vi "Laser 1 FP handler L3.vi"(5 "VISA Resource":T3[](array[typedef]), 6 "Numeric":dbl[](array[numeric]), 7 "FP Ops":T1, 8 "Error in":errorcluster caption="Error in (no error)", 9 "Boolean":bool[](array[boolean]), 10 "I/p string(s)":string[](array[string]), 11 "UI elements cluster":T2) -> (0 "Error out":errorcluster, 2 "Read Wavelength":dbl, 3 "Ls1 User Controls 2":T4)   [LabVIEW 2020]
uses:
  Type Defs/Ls1 User Controls.ctl
  Serial Comms/Visa resource.ctl
  Typedefs/UI ctrl refs cluster.ctl
  Typedefs/Laser control knob.ctl
  Typedefs/Frame Size.ctl
  Typedefs/Plane Mode.ctl
  Typedefs/PMT control knob.ctl
  Typedefs/XY Stage_Move.ctl
  Typedefs/test_fpga_control.ctl
  Acquisition/Typedefs/Ref DAQ Param.ctl
  User Interface/Misc/Experiment Type.ctl
  User Interface/Misc/Biology Information.ctl
  Type Defs/Ls1 User Ops.ctl
panel:
  out "Array":errorcluster[](array[cluster])
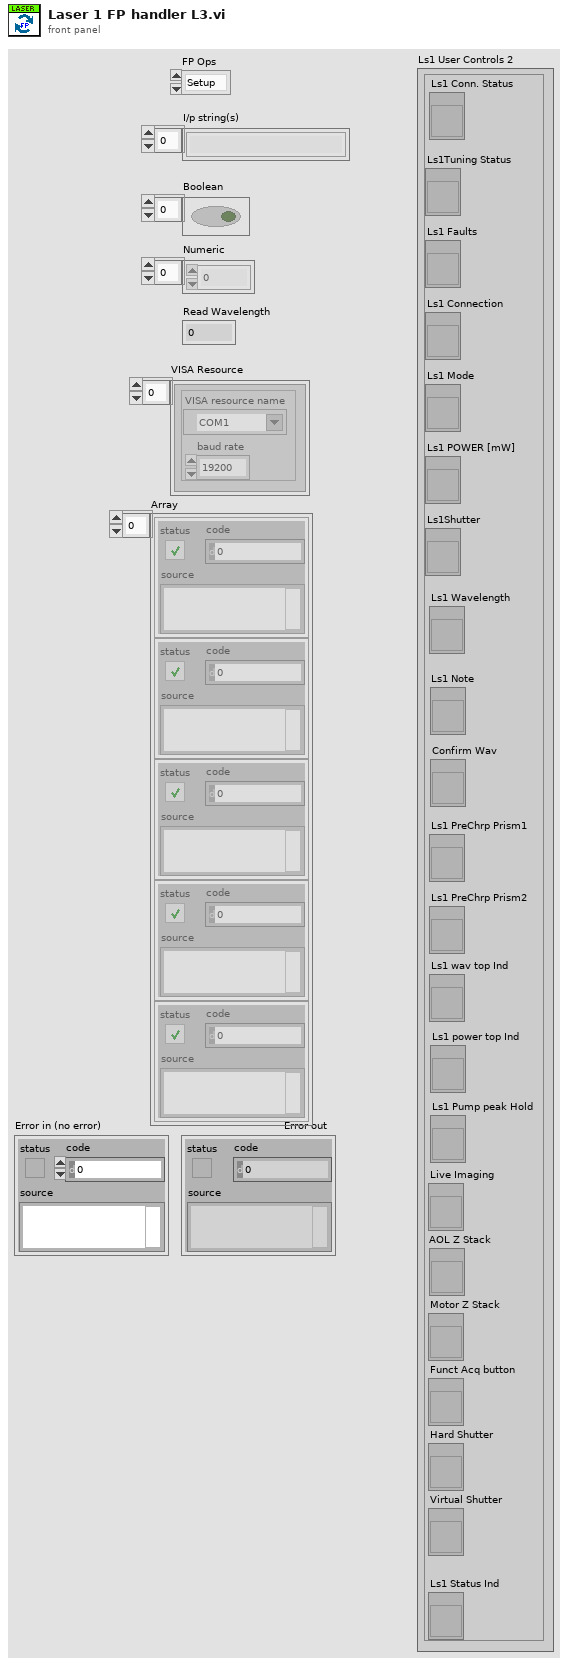
[diagram p1: front panel]
types:
  T1 = typedef "Ls1 User Ops.ctl" = enum16{"Setup", "Initialise", "Disable Controls", "Enable Controls", "Update Connection Info", "Update Laser Warning", "Update Laser status", "Update Laser status - sel", "Update Laser Wav.", "Update Laser Power", "Update prechiper settings", "Update Laser Note", "Update Shutter Status", "Close"}
  T2 = typedef "UI ctrl refs cluster.ctl" = cluster{"Top level VI path":path, "Top level VI ref":refnum<vi>, "User menu ref":refnum<k9>, "Sub Panel control":refnum<vi>, "Imaging Param Tab":refnum<vi>, "Occurrence-Start drivers":refnum<k4>, "Occurrence-Speed logging initialised":refnum<k4>, "Occurrence-XYZ stage initialised":refnum<k4>, "Exit button":refnum<vi>, "Status ind":refnum<vi>, "Set as origin":refnum<vi>, "Speed Logging":refnum<vi>, "Time Lapse":refnum<vi>, "Live Imaging":refnum<vi>, "AOL Z Stack":refnum<vi>, "Motor Z Stack":refnum<vi>, "Funct Acq button":refnum<vi>, "Hard Shutter":refnum<vi>, "Virtual Shutter":refnum<vi>, "Laser Power":refnum<vi>, "AOL Mode":refnum<vi>, "Frame Size":refnum<vi>, "Field of View":refnum<vi>, "Dwell Time":refnum<vi>, "Zoom":refnum<vi>, "AOL Z":refnum<vi>, "Objective":refnum<vi>, "Axis":refnum<vi>, "Paths & Names":refnum<vi>, "Experiment folder path (ind.)":refnum<vi>, "Last State (Ind.)":refnum<vi>, "Averages":refnum<vi>, "Angle (degrees)":refnum<vi>, "X centre":refnum<vi>, "Y centre":refnum<vi>, "Plane Mode":refnum<vi>, "# Planes":refnum<vi>, "Z Start":refnum<vi>, "Z Stop":refnum<vi>, "Z Step":refnum<vi>, "PMT 1":refnum<vi>, "PMT 2":refnum<vi>, "Stage XYZ Position":refnum<vi>, "Pockels@Z Start":refnum<vi>, "Pockels@Z Stop":refnum<vi>, "Obtain Z Start":refnum<vi>, "Obtain Z Stop":refnum<vi>, "Live stim.trig.period":refnum<vi>, "Live stim.trig.enable":refnum<vi>, "Movement Correction":refnum<vi>, "Load Reference Image":refnum<vi>, "XY Stage Move":refnum<vi>, "MovCor Cluster":refnum<vi>, "RefDAQParam":refnum<vi>, "Funct. Acq. Pockels Modulation":refnum<vi>, "Ref Laser Power":refnum<vi>, "Enable Video Recording":refnum<vi>, "Video Record-Live Imaging":refnum<vi>, "Video Record-Funct acq":refnum<vi>, "Reference Source":refnum<vi>, "AOL Z-stack Chirps Ready (ind)":refnum<vi>, "Target time between mov.cor. ref triggers (ms)":refnum<vi>, "Funct. Acq. Ref frame save":refnum<vi>, "Tracking button":refnum<vi>, "Show ref plots window":refnum<vi>, "Center freq ind (nm)":refnum<vi>, "Pickup mode (ind)":refnum<vi>, "Logging queue (ind)":refnum<vi>, "Back aperture power (ind.)":refnum<vi>, "Power after objective (ind.)":refnum<vi>, "Switch user":refnum<vi>, "Ls1 Conn. Status":refnum<vi>, "Ls1Tuning Status":refnum<vi>, "Ls1 Faults":refnum<vi>, "Ls1 Connection":refnum<vi>, "Ls1 Mode":refnum<vi>, "Ls1 POWER [mW]":refnum<vi>, "Ls1Shutter":refnum<vi>, "Ls1 Wavelength":refnum<vi>, "Ls1 Note":refnum<vi>, "Ls1 Confirm Wav":refnum<vi>, "Ls1 PreChrp Prism1":refnum<vi>, "Ls1 PreChrp Prism2":refnum<vi>, "Ls1 wav top Ind":refnum<vi>, "Ls1 power top Ind":refnum<vi>, "Ls1 Pump peak Hold":refnum<vi>, "Ls1 Status Ind":refnum<vi>, "Ls1 wav cancel":refnum<vi>, "Experiment Type":refnum<vi>, "Biology Information":refnum<vi>, "Camera recording status":refnum<vi>, "Optimise Obj. Pos.":refnum<vi>}
  T3 = typedef "Visa resource.ctl" = cluster{"VISA resource name":refnum<visa-resource-name>, "baud rate":u32}
  T4 = typedef "Ls1 User Controls.ctl" = cluster{"Ls1 Conn. Status":refnum<vi>, "Ls1Tuning Status":refnum<vi>, "Ls1 Faults":refnum<vi>, "Ls1 Connection":refnum<vi>, "Ls1 Mode":refnum<vi>, "Ls1 POWER [mW]":refnum<vi>, "Ls1Shutter":refnum<vi>, "Ls1 Wavelength":refnum<vi>, "Ls1 Note":refnum<vi>, "Confirm Wav":refnum<vi>, "Ls1 PreChrp Prism1":refnum<vi>, "Ls1 PreChrp Prism2":refnum<vi>, "Ls1 wav top Ind":refnum<vi>, "Ls1 power top Ind":refnum<vi>, "Ls1 Pump peak Hold":refnum<vi>, "Live Imaging":refnum<vi>, "AOL Z Stack":refnum<vi>, "Motor Z Stack":refnum<vi>, "Funct Acq button":refnum<vi>, "Hard Shutter":refnum<vi>, "Virtual Shutter":refnum<vi>, "Ls1 Status Ind":refnum<vi>}
  T5 = enum8{"Enabled", "Disabled", "Disabled and Grayed Out"}
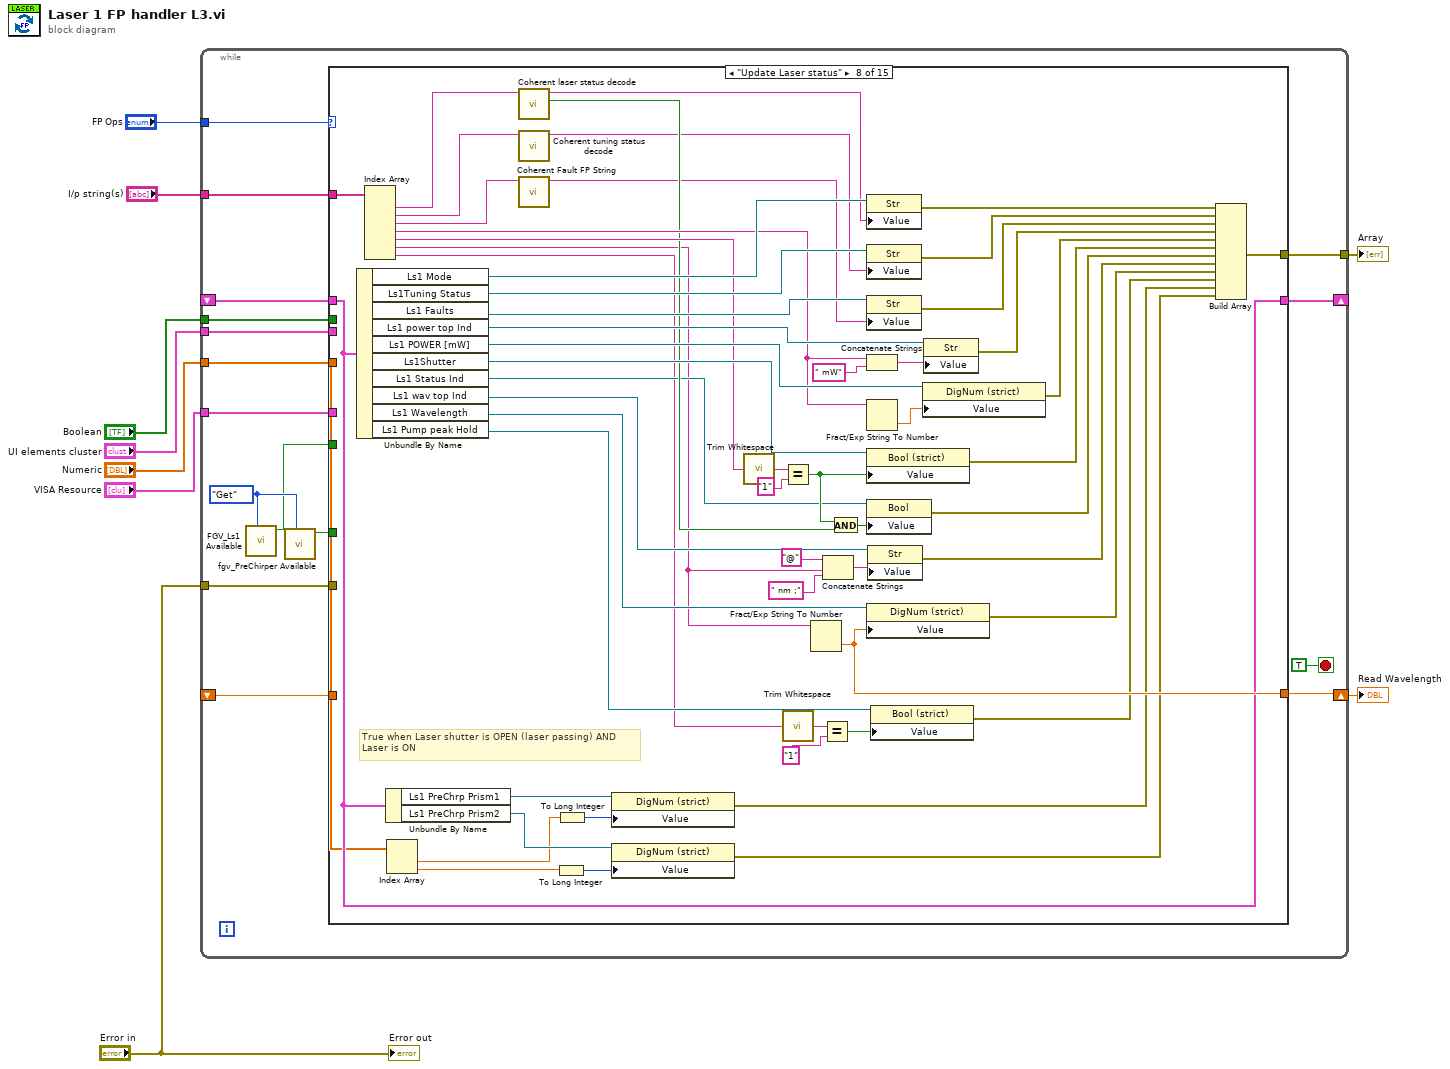
[diagram p0: block diagram]
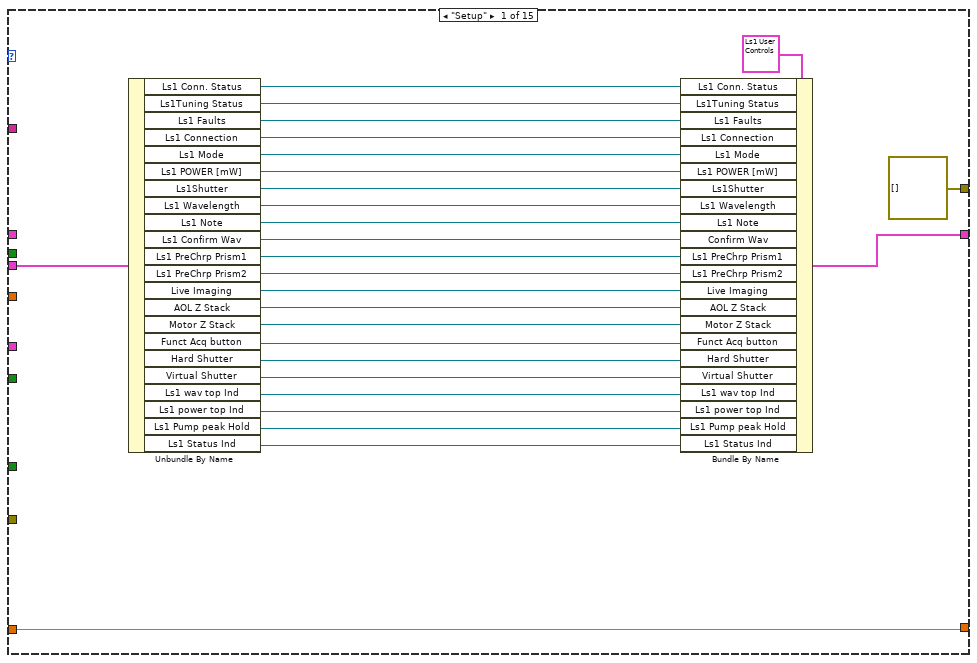
[diagram p2: hidden frame]
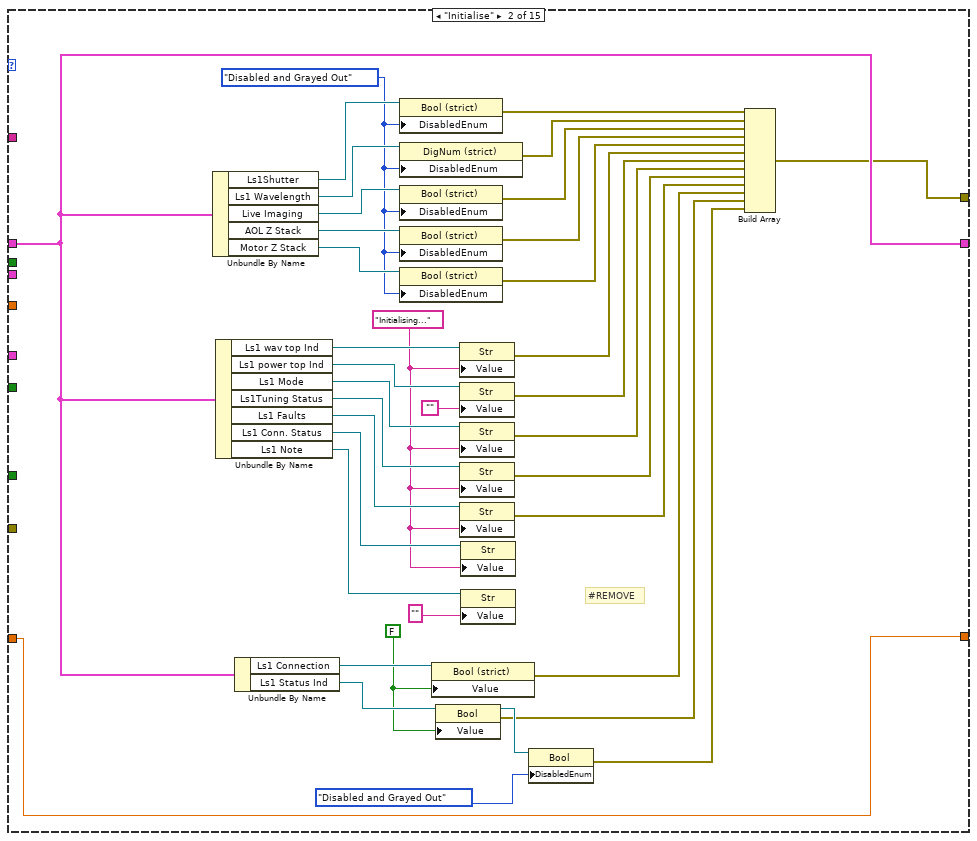
[diagram p3: hidden frame]
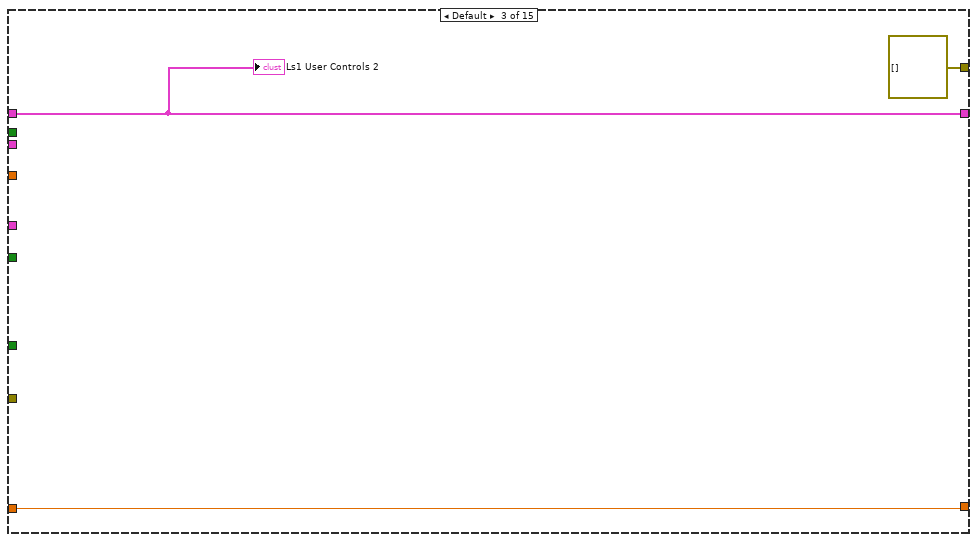
[diagram p4: hidden frame]
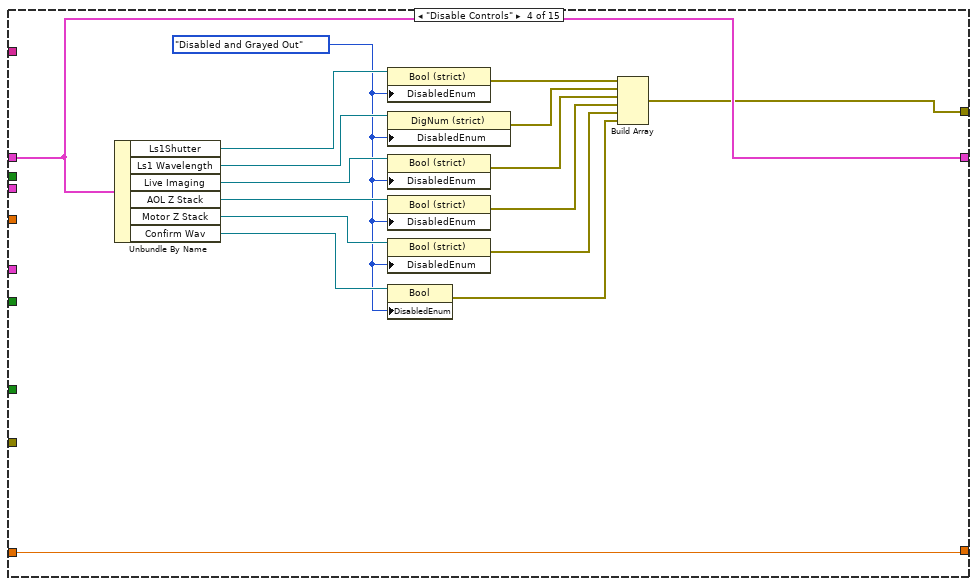
[diagram p5: hidden frame]
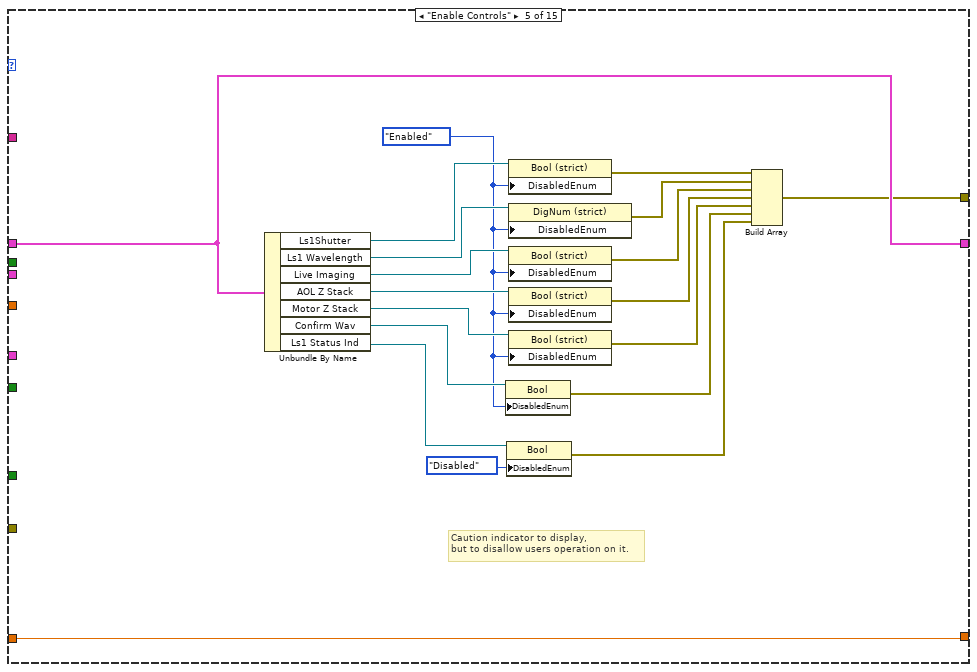
[diagram p6: hidden frame]
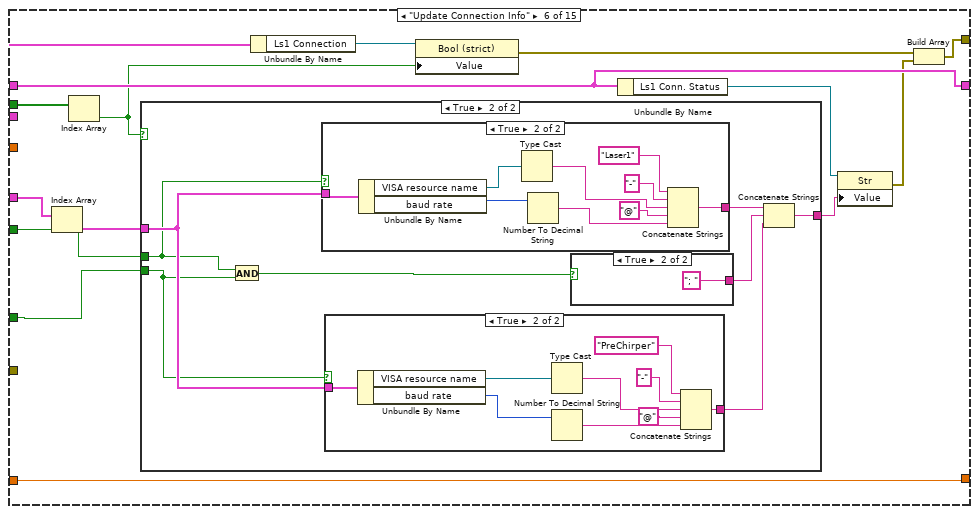
[diagram p7: hidden frame]
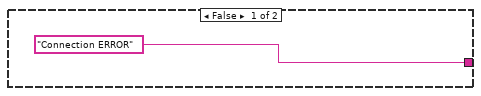
[diagram p8: hidden frame]
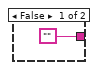
[diagram p9: hidden frame]
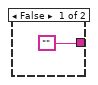
[diagram p10: hidden frame]
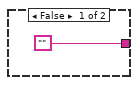
[diagram p11: hidden frame]
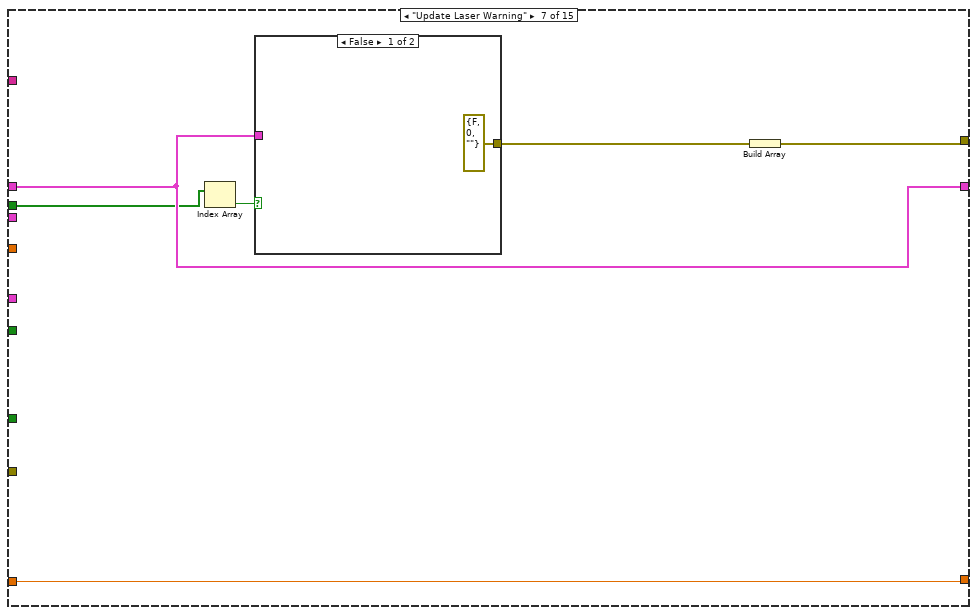
[diagram p12: hidden frame]
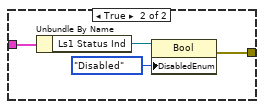
[diagram p13: hidden frame]
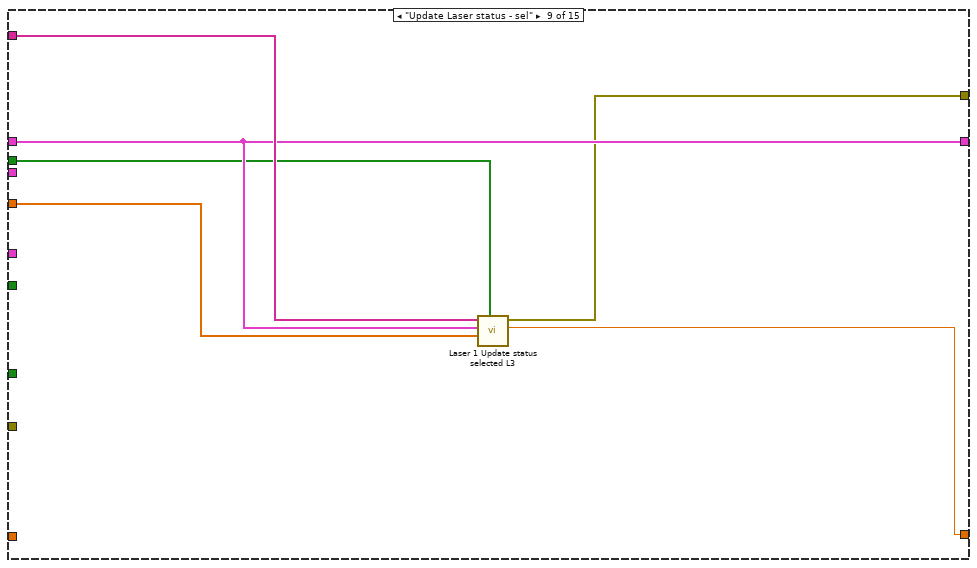
[diagram p14: hidden frame]
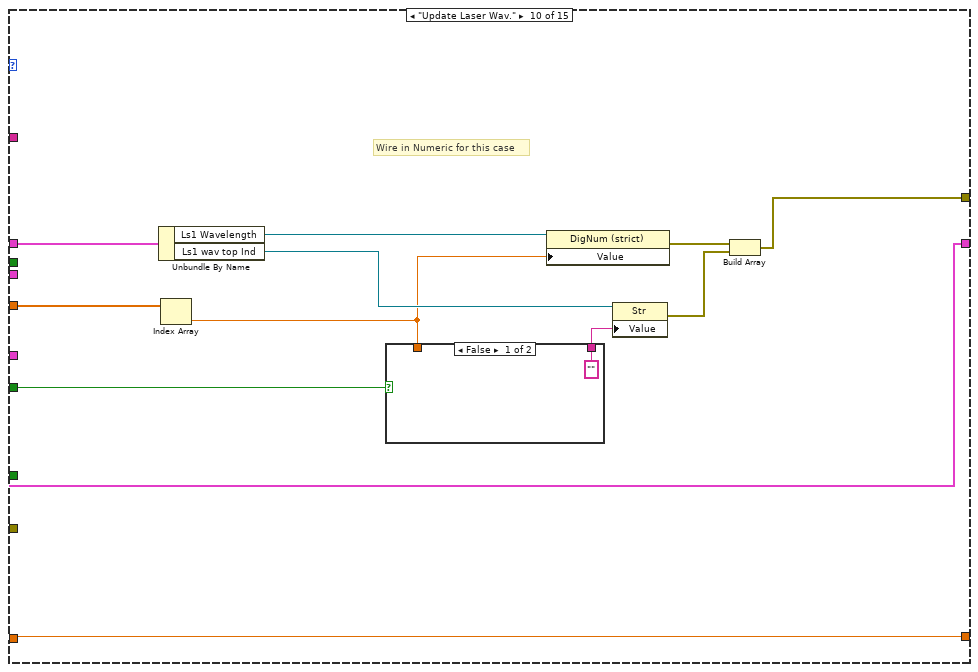
[diagram p15: hidden frame]
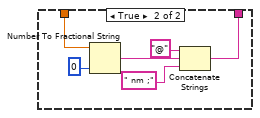
[diagram p16: hidden frame]
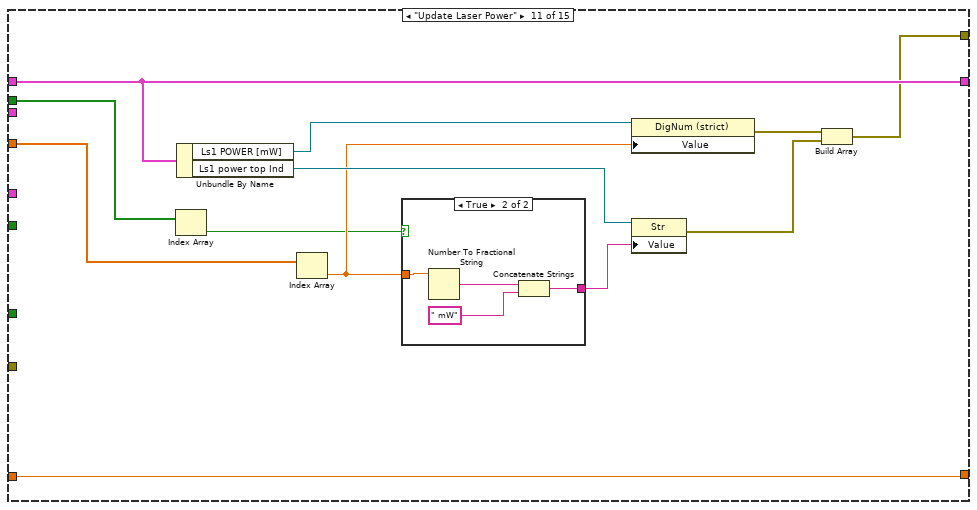
[diagram p17: hidden frame]
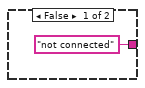
[diagram p18: hidden frame]
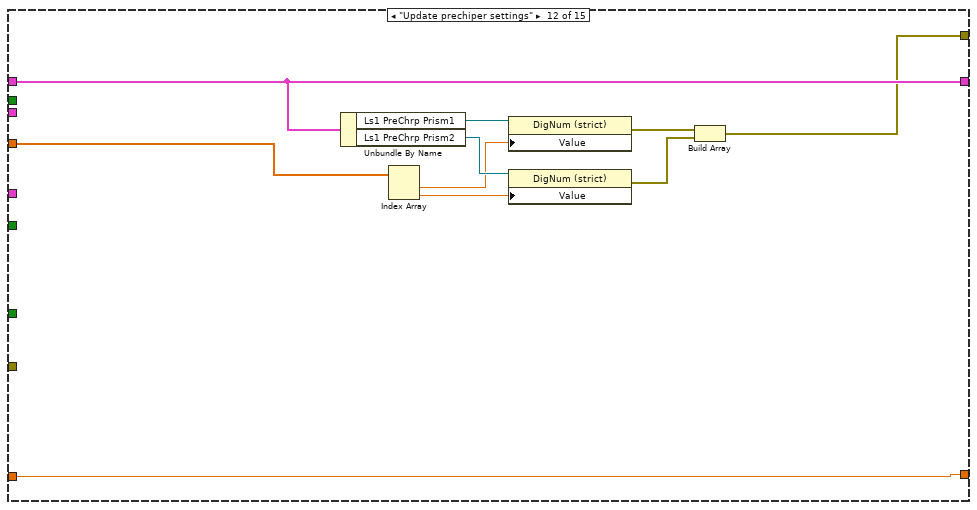
[diagram p19: hidden frame]
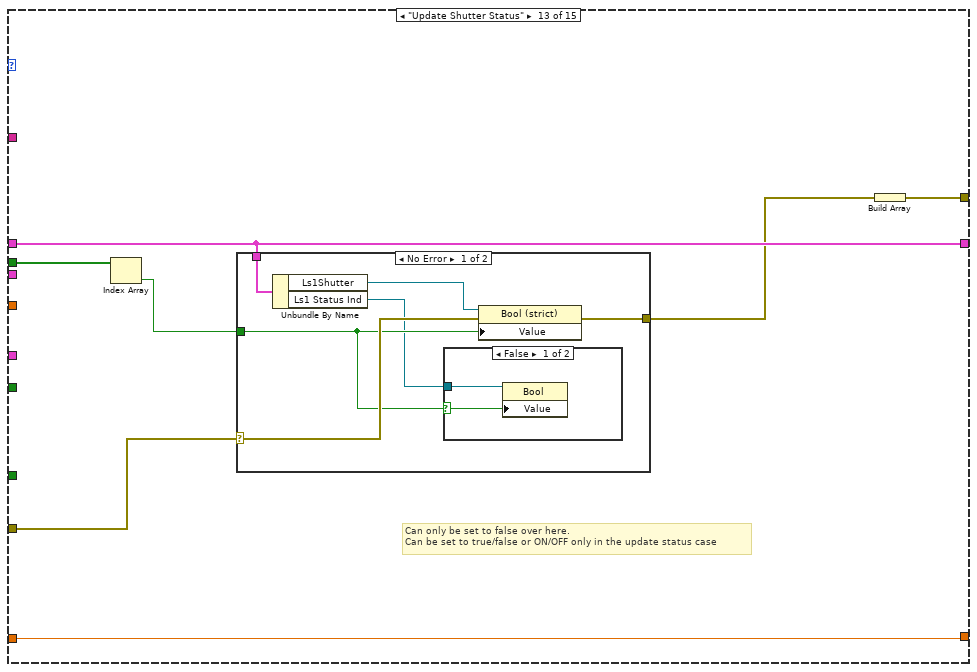
[diagram p20: hidden frame]
diagram:
  n1 = while {
    tunnel: "FP Ops" -> [w25]
    tunnel: "Boolean" -> [w23]
    tunnel: "I/p string(s)" -> [w22]
    tunnel: "VISA Resource" -> [w21]
    tunnel: "Numeric" -> [w20]
    shift-right: [w17] -> _
    shift-left: _ -> [w24]
    tunnel: "UI elements cluster" -> [w18]
    shift-right: [w16] -> w3
    shift-left: _ -> [w15]
    tunnel: "Error in" -> [w14]
    tunnel: [w13] -> w1
    stop <- TRUE stop-if-true
    w12 = enum16{"Get", "Set"}."Get" ("FGV Actions")
    n2 = call "FGV_Ls1 Available.vi"("FGV Actions"=w12) -> ("Laser Available ? OUT"=w10:bool)  [unwired: 9 in, 1 out]
    n3 = call "fgv_PreChirper Available.vi"("FGV Actions"=w12) -> ("PreChirper Available ? OUT"=w11:bool)  [unwired: 9 in, 1 out]
    n4 = case shown="\"Update Laser status\"" w25 {
      tunnel: w24 -> [_ w78 w92 w103 w122 w140 w178 w207 w244 w257 w276 w291 w298 w314 w338]
      tunnel: w22 -> [_ _ _ _ _ _ _ w237 w246 _ _ _ _ w312 _]
      tunnel: w23 -> [_ _ _ _ _ w135 w177 _ w241 _ w271 _ w297 _ _]
      tunnel: w20 -> [_ _ _ _ _ _ _ w206 w243 w255 w274 w288 _ _ _]
      tunnel: w21 -> [_ _ _ _ _ w137 _ _ _ _ _ _ _ _ _]
      tunnel: w18 -> [w33 _ _ _ _ _ _ _ _ _ _ _ _ _ _]
      tunnel: [w43 w78 w92 w103 w122 w140 w178 w207 w244 w257 w276 w291 w298 w314 w338] -> w17
      tunnel: [w29 w72 w91 w102 w121 w133 w175 w210 w245 w254 w268 w285 w295 w310 w337] -> w16
      tunnel: w15 -> [w29 w72 w91 w102 w121 w133 w175 _ _ w254 w268 w285 w295 w310 w337]
      tunnel: w14 -> [_ _ _ _ _ _ _ _ _ _ _ _ w294 w309 _]
      tunnel: [errorcluster[] [] w58 errorcluster[] [] w96 w115 w130 w173 w191 w242 w248 w265 w282 w293 w308 w325] -> w13
      tunnel: w10 -> [_ _ _ _ _ w129 _ _ _ w247 _ _ _ _ w315]
      tunnel: w11 -> [_ _ _ _ _ w128 _ _ _ _ _ _ _ _ _]
      frame "Setup" {
        n5 = Unbundle By Name(w33) -> ("Ls1 Conn. Status"=w34:refnum<vi>, "Ls1Tuning Status"=w36:refnum<vi>, "Ls1 Faults"=w51:refnum<vi>, "Ls1 Connection"=w50:refnum<vi>, "Ls1 Mode"=w49:refnum<vi>, "Ls1 POWER [mW]"=w48:refnum<vi>, "Ls1Shutter"=w47:refnum<vi>, "Ls1 Wavelength"=w46:refnum<vi>, "Ls1 Note"=w45:refnum<vi>, "Ls1 Confirm Wav"=w35:refnum<vi>, "Ls1 PreChrp Prism1"=w27:refnum<vi>, "Ls1 PreChrp Prism2"=w44:refnum<vi>, "Live Imaging"=w42:refnum<vi>, "AOL Z Stack"=w41:refnum<vi>, "Motor Z Stack"=w40:refnum<vi>, "Funct Acq button"=w39:refnum<vi>, "Hard Shutter"=w38:refnum<vi>, "Virtual Shutter"=w37:refnum<vi>, "Ls1 wav top Ind"=w32:refnum<vi>, "Ls1 power top Ind"=w31:refnum<vi>, "Ls1 Pump peak Hold"=w30:refnum<vi>, "Ls1 Status Ind"=w28:refnum<vi>)
        n6 = Bundle By Name(cluster=T4 {"Ls1 Conn. Status"=refnum, "Ls1Tuning Status"=refnum, "Ls1 Faults"=refnum, "Ls1 Connection"=refnum, "Ls1 Mode"=refnum, "Ls1 POWER [mW]"=refnum, "Ls1Shutter"=refnum, "Ls1 Wavelength"=refnum, "Ls1 Note"=refnum, "Confirm Wav"=refnum, "Ls1 PreChrp Prism1"=refnum, "Ls1 PreChrp Prism2"=refnum, "Ls1 wav top Ind"=refnum, "Ls1 power top Ind"=refnum, "Ls1 Pump peak Hold"=refnum, "Live Imaging"=refnum, "AOL Z Stack"=refnum, "Motor Z Stack"=refnum, "Funct Acq button"=refnum, "Hard Shutter"=refnum, "Virtual Shutter"=refnum, "Ls1 Status Ind"=refnum} ("Ls1 User Controls"), "Ls1 Conn. Status"=w34, "Ls1Tuning Status"=w36, "Ls1 Faults"=w51, "Ls1 Connection"=w50, "Ls1 Mode"=w49, "Ls1 POWER [mW]"=w48, "Ls1Shutter"=w47, "Ls1 Wavelength"=w46, "Ls1 Note"=w45, "Confirm Wav"=w35, "Ls1 PreChrp Prism1"=w27, "Ls1 PreChrp Prism2"=w44, "Live Imaging"=w42, "AOL Z Stack"=w41, "Motor Z Stack"=w40, "Funct Acq button"=w39, "Hard Shutter"=w38, "Virtual Shutter"=w37, "Ls1 wav top Ind"=w32, "Ls1 power top Ind"=w31, "Ls1 Pump peak Hold"=w30, "Ls1 Status Ind"=w28) -> (w43:T4)
      }
      frame "Initialise" {
        w75 = FALSE ("Value")
        w56 = "Initialising..." ("Value")
        w84 = T5."Disabled and Grayed Out" ("Disabled")
        # "#REMOVE"
        n7 = Unbundle By Name(w78) -> ("Ls1Shutter"=w88:refnum<vi>, "Ls1 Wavelength"=w89:refnum<vi>, "Live Imaging"=w87:refnum<vi>, "AOL Z Stack"=w86:refnum<vi>, "Motor Z Stack"=w85:refnum<vi>)
        n8 = Unbundle By Name(w78) -> ("Ls1 wav top Ind"=w83:refnum<vi>, "Ls1 power top Ind"=w82:refnum<vi>, "Ls1 Mode"=w81:refnum<vi>, "Ls1Tuning Status"=w80:refnum<vi>, "Ls1 Faults"=w79:refnum<vi>, "Ls1 Conn. Status"=w57:refnum<vi>, "Ls1 Note"=w55:refnum<vi>)
        n9 = Unbundle By Name(w78) -> ("Ls1 Connection"=w77:refnum<vi>, "Ls1 Status Ind"=w76:refnum<vi>)
        n10 = property class="Bool (strict)"(reference=w88, "DisabledEnum"=w84) -> (error out=w71:errorcluster)  [unwired: 1 in, 1 out]
        n11 = property class="DigNum (strict)"(reference=w89, "DisabledEnum"=w84) -> (error out=w70:errorcluster)  [unwired: 1 in, 1 out]
        n12 = property class="Bool (strict)"(reference=w87, "DisabledEnum"=w84) -> (error out=w69:errorcluster)  [unwired: 1 in, 1 out]
        n13 = property class="Bool (strict)"(reference=w86, "DisabledEnum"=w84) -> (error out=w68:errorcluster)  [unwired: 1 in, 1 out]
        n14 = property class="Bool (strict)"(reference=w85, "DisabledEnum"=w84) -> (error out=w67:errorcluster)  [unwired: 1 in, 1 out]
        n15 = property class="Bool (strict)"(reference=w77, "Value"=w75) -> (error out=w61:errorcluster)  [unwired: 1 in, 1 out]
        n16 = property class="Bool"(reference=w76, "Value"=w75) -> (reference out=w74:refnum<vi>, error out=w60:errorcluster)  [unwired: 1 in]
        n17 = property class="Str"(reference=w83, "Value"=w56) -> (error out=w66:errorcluster)  [unwired: 1 in, 1 out]
        n18 = property class="Str"(reference=w82, "Value"="") -> (error out=w65:errorcluster)  [unwired: 1 in, 1 out]
        n19 = property class="Str"(reference=w81, "Value"=w56) -> (error out=w64:errorcluster)  [unwired: 1 in, 1 out]
        n20 = property class="Str"(reference=w80, "Value"=w56) -> (error out=w63:errorcluster)  [unwired: 1 in, 1 out]
        n21 = property class="Str"(reference=w79, "Value"=w56) -> (error out=w62:errorcluster)  [unwired: 1 in, 1 out]
        n22 = property class="Str"(reference=w57, "Value"=w56) -> ()  [unwired: 1 in, 2 out]
        n23 = property class="Str"(reference=w55, "Value"="") -> ()  [unwired: 1 in, 2 out]
        n24 = property class="Bool"(reference=w74, "DisabledEnum"=T5."Disabled and Grayed Out" ("Disabled")) -> (error out=w59:errorcluster)  [unwired: 1 in, 1 out]
        n25 = Build Array(w71, w70, w69, w68, w67, w66, w65, w64, w63, w62, w61, w60, w59) -> (w58:errorcluster[])
      }
      frame Default {
        "Ls1 User Controls 2" <- w92
      }
      frame "Disable Controls" {
        w94 = T5."Disabled and Grayed Out" ("Disabled")
        n26 = Unbundle By Name(w103) -> ("Ls1Shutter"=w107:refnum<vi>, "Ls1 Wavelength"=w108:refnum<vi>, "Live Imaging"=w106:refnum<vi>, "AOL Z Stack"=w105:refnum<vi>, "Motor Z Stack"=w104:refnum<vi>, "Confirm Wav"=w95:refnum<vi>)
        n27 = property class="Bool (strict)"(reference=w107, "DisabledEnum"=w94) -> (error out=w101:errorcluster)  [unwired: 1 in, 1 out]
        n28 = property class="DigNum (strict)"(reference=w108, "DisabledEnum"=w94) -> (error out=w100:errorcluster)  [unwired: 1 in, 1 out]
        n29 = property class="Bool (strict)"(reference=w106, "DisabledEnum"=w94) -> (error out=w99:errorcluster)  [unwired: 1 in, 1 out]
        n30 = property class="Bool (strict)"(reference=w105, "DisabledEnum"=w94) -> (error out=w98:errorcluster)  [unwired: 1 in, 1 out]
        n31 = property class="Bool (strict)"(reference=w104, "DisabledEnum"=w94) -> (error out=w97:errorcluster)  [unwired: 1 in, 1 out]
        n32 = property class="Bool"(reference=w95, "DisabledEnum"=w94) -> (error out=w93:errorcluster)  [unwired: 1 in, 1 out]
        n33 = Build Array(w101, w100, w99, w98, w97, w93) -> (w96:errorcluster[])
      }
      frame "Enable Controls" {
        w113 = T5."Enabled" ("Disabled")
        # "Caution indicator to display,\nbut to disallow users operation on it."
        n34 = Unbundle By Name(w122) -> ("Ls1Shutter"=w126:refnum<vi>, "Ls1 Wavelength"=w127:refnum<vi>, "Live Imaging"=w125:refnum<vi>, "AOL Z Stack"=w124:refnum<vi>, "Motor Z Stack"=w123:refnum<vi>, "Confirm Wav"=w114:refnum<vi>, "Ls1 Status Ind"=w111:refnum<vi>)
        n35 = property class="Bool"(reference=w114, "DisabledEnum"=w113) -> (error out=w112:errorcluster)  [unwired: 1 in, 1 out]
        n36 = property class="Bool"(reference=w111, "DisabledEnum"=T5."Disabled" ("Disabled")) -> (error out=w109:errorcluster)  [unwired: 1 in, 1 out]
        n37 = property class="Bool (strict)"(reference=w126, "DisabledEnum"=w113) -> (error out=w120:errorcluster)  [unwired: 1 in, 1 out]
        n38 = property class="DigNum (strict)"(reference=w127, "DisabledEnum"=w113) -> (error out=w119:errorcluster)  [unwired: 1 in, 1 out]
        n39 = property class="Bool (strict)"(reference=w125, "DisabledEnum"=w113) -> (error out=w118:errorcluster)  [unwired: 1 in, 1 out]
        n40 = property class="Bool (strict)"(reference=w124, "DisabledEnum"=w113) -> (error out=w117:errorcluster)  [unwired: 1 in, 1 out]
        n41 = property class="Bool (strict)"(reference=w123, "DisabledEnum"=w113) -> (error out=w116:errorcluster)  [unwired: 1 in, 1 out]
        n42 = Build Array(w120, w119, w118, w117, w116, w112, w109) -> (w115:errorcluster[])
      }
      frame "Update Connection Info" {
        n43 = Index Array(array=w137) -> (element=w138:T3)  [unwired: 1 in]
        n44 = Index Array(array=w135) -> (element=w134:bool)  [unwired: 1 in]
        n45 = case shown="True" w134 {
          tunnel: w138 -> [_ w147]
          tunnel: ["Connection ERROR" w146] -> w136
          tunnel: w129 -> [_ w145]
          tunnel: w128 -> [_ w144]
          frame False {
          }
          frame True {
            n46 = And(x=w145, y=w144) -> (x .and. y?=w143:bool)
            n47 = case shown="True" w145 {
              tunnel: ["" w165] -> w150
              tunnel: w147 -> [_ w164]
              frame False {
              }
              frame True {
                n48 = Unbundle By Name(w164) -> ("VISA resource name"=w172:refnum<visa-resource-name>, "baud rate"=w171:u32)
                n49 = Type Cast(x=w172) -> (*(type *) &x=w167:string)  [unwired: 1 in]
                n50 = Number To Decimal String(number=w171) -> (decimal integer string=w166:string)  [unwired: 1 in]
                n51 = Concatenate Strings("Laser1", "-" ("string"), w167, "@" ("string"), w166) -> (w165:string)
              }
            }
            n52 = case shown="True" w144 {
              tunnel: ["" w156] -> w149
              tunnel: w147 -> [_ w154]
              frame False {
              }
              frame True {
                n53 = Unbundle By Name(w154) -> ("VISA resource name"=w157:refnum<visa-resource-name>, "baud rate"=w155:u32)
                n54 = Type Cast(x=w157) -> (*(type *) &x=w159:string)  [unwired: 1 in]
                n55 = Number To Decimal String(number=w155) -> (decimal integer string=w158:string)  [unwired: 1 in]
                n56 = Concatenate Strings("PreChirper", "-" ("string"), w159, "@" ("string"), w158) -> (w156:string)
              }
            }
            n57 = case shown="True" w143 {
              tunnel: ["" "; "] -> w148
              frame False {
              }
              frame True {
              }
            }
            n58 = Concatenate Strings(w150, w148, w149) -> (w146:string)
          }
        }
        n59 = Unbundle By Name(w140) -> ("Ls1 Connection"=w139:refnum<vi>)
        n60 = property class="Bool (strict)"(reference=w139, "Value"=w134) -> (error out=w131:errorcluster)  [unwired: 1 in, 1 out]
        n61 = Unbundle By Name(w140) -> ("Ls1 Conn. Status"=w141:refnum<vi>)
        n62 = property class="Str"(reference=w141, "Value"=w136) -> (error out=w132:errorcluster)  [unwired: 1 in, 1 out]
        n63 = Build Array(w131, w132) -> (w130:errorcluster[])
      }
      frame "Update Laser Warning" {
        n64 = Index Array(array=w177) -> (element=w176:bool)  [unwired: 1 in]
        n65 = case shown="False" w176 {
          tunnel: w178 -> [_ w183]
          tunnel: [errorcluster {"status"=FALSE, "code"=0, "source"=""} ("error out") w180] -> w174
          frame False {
          }
          frame True {
            n66 = Unbundle By Name(w183) -> ("Ls1 Status Ind"=w182:refnum<vi>)
            n67 = property class="Bool"(reference=w182, "DisabledEnum"=T5."Disabled" ("Disabled")) -> (error out=w180:errorcluster)  [unwired: 1 in, 1 out]
          }
        }
        n68 = Build Array(w174) -> (w173:errorcluster[])
      }
      frame "Update Laser status" {
        # "True when Laser shutter is OPEN (laser passing) AND\nLaser is ON"
        n69 = Unbundle By Name(w207) -> ("Ls1 Mode"=w240:refnum<vi>, "Ls1Tuning Status"=w239:refnum<vi>, "Ls1 Faults"=w238:refnum<vi>, "Ls1 power top Ind"=w236:refnum<vi>, "Ls1 POWER [mW]"=w235:refnum<vi>, "Ls1Shutter"=w230:refnum<vi>, "Ls1 Status Ind"=w221:refnum<vi>, "Ls1 wav top Ind"=w218:refnum<vi>, "Ls1 Wavelength"=w217:refnum<vi>, "Ls1 Pump peak Hold"=w213:refnum<vi>)
        n70 = Index Array(array=w237) -> (element #1=w226:string, element #2=w187:string, element #3=w185:string, element #4=w233:string, element #5=w229:string, element #6=w216:string, element #7=w211:string)  [unwired: 7 in]
        n71 = Unbundle By Name(w207) -> ("Ls1 PreChrp Prism1"=w209:refnum<vi>, "Ls1 PreChrp Prism2"=w208:refnum<vi>)
        n72 = Index Array(array=w206) -> (element #1=w204:dbl, element #2=w202:dbl)  [unwired: 2 in]
        n73 = call "Coherent laser status decode.vi"("I/p String"=w226) -> ("Boolean"=w222:bool, "String"=w225:string)  [unwired: 9 in]
        n74 = call "Coherent tuning status decode.vi"("I/p String"=w187) -> ("O/P String"=w186:string)  [unwired: 10 in]
        n75 = call "Coherent Fault FP String.vi"("I/p String"=w185) -> ("O/P String"=w184:string)  [unwired: 10 in]
        n76 = To Long Integer(number=w202) -> (32bit integer=w203:i32)
        n77 = To Long Integer(number=w204) -> (32bit integer=w205:i32)
        n78 = property class="DigNum (strict)"(reference=w209, "Value"=w205) -> (error out=w190:errorcluster)  [unwired: 1 in, 1 out]
        n79 = property class="DigNum (strict)"(reference=w208, "Value"=w203) -> (error out=w189:errorcluster)  [unwired: 1 in, 1 out]
        n80 = call <vilib>:"Trim Whitespace.vi"("string"=w229) -> ("trimmed string"=w228:string)  [unwired: 1 in]
        n81 = Equal?(x=w228, y="1") -> (x = y?=w223:bool)
        n82 = call <vilib>:"Trim Whitespace.vi"("string"=w211) -> ("trimmed string"=w215:string)  [unwired: 1 in]
        n83 = Fract/Exp String To Number(string=w216) -> (number=w210:dbl)  [unwired: 3 in, 1 out]
        n84 = Equal?(x=w215, y="1") -> (x = y?=w212:bool)
        n85 = Concatenate Strings("@" ("string"), w216, " nm ;" ("string")) -> (w219:string)
        n86 = And(x=w223, y=w222) -> (x .and. y?=w224:bool)
        n87 = property class="Str"(reference=w240, "Value"=w225) -> (error out=w201:errorcluster)  [unwired: 1 in, 1 out]
        n88 = property class="Str"(reference=w239, "Value"=w186) -> (error out=w200:errorcluster)  [unwired: 1 in, 1 out]
        n89 = property class="Str"(reference=w238, "Value"=w184) -> (error out=w199:errorcluster)  [unwired: 1 in, 1 out]
        n90 = Concatenate Strings(w233, " mW" ("string")) -> (w231:string)
        n91 = Fract/Exp String To Number(string=w233) -> (number=w234:dbl)  [unwired: 3 in, 1 out]
        n92 = property class="Bool (strict)"(reference=w230, "Value"=w223) -> (error out=w196:errorcluster)  [unwired: 1 in, 1 out]
        n93 = property class="Bool"(reference=w221, "Value"=w224) -> (error out=w195:errorcluster)  [unwired: 1 in, 1 out]
        n94 = property class="DigNum (strict)"(reference=w217, "Value"=w210) -> (error out=w193:errorcluster)  [unwired: 1 in, 1 out]
        n95 = property class="Str"(reference=w218, "Value"=w219) -> (error out=w194:errorcluster)  [unwired: 1 in, 1 out]
        n96 = property class="Bool (strict)"(reference=w213, "Value"=w212) -> (error out=w192:errorcluster)  [unwired: 1 in, 1 out]
        n97 = property class="DigNum (strict)"(reference=w235, "Value"=w234) -> (error out=w197:errorcluster)  [unwired: 1 in, 1 out]
        n98 = property class="Str"(reference=w236, "Value"=w231) -> (error out=w198:errorcluster)  [unwired: 1 in, 1 out]
        n99 = Build Array(w201, w200, w199, w198, w197, w196, w195, w194, w193, w192, w190, w189) -> (w191:errorcluster[])
      }
      frame "Update Laser status - sel" {
        n100 = call "Laser 1 Update status selected L3.vi"("Array"=w241, "Numeric in"=w243, "Ls1 User Controls"=w244, "I/p string(s)"=w246) -> ("Numeric out"=w245:dbl, "Array"=w242:errorcluster[])  [unwired: 6 in]
      }
      frame "Update Laser Wav." {
        # "Wire in Numeric for this case"
        n101 = Unbundle By Name(w257) -> ("Ls1 Wavelength"=w256:refnum<vi>, "Ls1 wav top Ind"=w253:refnum<vi>)
        n102 = Index Array(array=w255) -> (element=w252:dbl)  [unwired: 1 in]
        n103 = case shown="False" w247 {
          tunnel: w252 -> [_ w264]
          tunnel: ["" w261] -> w251
          frame False {
          }
          frame True {
            n104 = Number To Fractional String(number=w264, precision (6)=i16 0) -> (F-format string=w263:string)  [unwired: 2 in]
            n105 = Concatenate Strings("@" ("string"), w263, " nm ;" ("string")) -> (w261:string)
          }
        }
        n106 = property class="DigNum (strict)"(reference=w256, "Value"=w252) -> (error out=w250:errorcluster)  [unwired: 1 in, 1 out]
        n107 = property class="Str"(reference=w253, "Value"=w251) -> (error out=w249:errorcluster)  [unwired: 1 in, 1 out]
        n108 = Build Array(w250, w249) -> (w248:errorcluster[])
      }
      frame "Update Laser Power" {
        n109 = Index Array(array=w271) -> (element=w270:bool)  [unwired: 1 in]
        n110 = Unbundle By Name(w276) -> ("Ls1 POWER [mW]"=w273:refnum<vi>, "Ls1 power top Ind"=w275:refnum<vi>)
        n111 = Index Array(array=w274) -> (element=w272:dbl)  [unwired: 1 in]
        n112 = case shown="True" w270 {
          tunnel: w272 -> [_ w279]
          tunnel: ["not connected" w278] -> w269
          frame False {
          }
          frame True {
            n113 = Number To Fractional String(number=w279) -> (F-format string=w281:string)  [unwired: 3 in]
            n114 = Concatenate Strings(w281, " mW" ("string")) -> (w278:string)
          }
        }
        n115 = property class="DigNum (strict)"(reference=w273, "Value"=w272) -> (error out=w267:errorcluster)  [unwired: 1 in, 1 out]
        n116 = property class="Str"(reference=w275, "Value"=w269) -> (error out=w266:errorcluster)  [unwired: 1 in, 1 out]
        n117 = Build Array(w267, w266) -> (w265:errorcluster[])
      }
      frame "Update prechiper settings" {
        n118 = Unbundle By Name(w291) -> ("Ls1 PreChrp Prism1"=w290:refnum<vi>, "Ls1 PreChrp Prism2"=w289:refnum<vi>)
        n119 = Index Array(array=w288) -> (element #1=w287:dbl, element #2=w286:dbl)  [unwired: 2 in]
        n120 = property class="DigNum (strict)"(reference=w290, "Value"=w287) -> (error out=w284:errorcluster)  [unwired: 1 in, 1 out]
        n121 = property class="DigNum (strict)"(reference=w289, "Value"=w286) -> (error out=w283:errorcluster)  [unwired: 1 in, 1 out]
        n122 = Build Array(w284, w283) -> (w282:errorcluster[])
      }
      frame "Update Shutter Status" {
        # "Can only be set to false over here.\nCan be set to true/false or ON/OFF only in the update status case"
        n123 = Index Array(array=w297) -> (element=w296:bool)  [unwired: 1 in]
        n124 = case shown="No Error" w294 {
          selector: w294 -> [w302 w307]
          tunnel: w298 -> [w303 _]
          tunnel: w296 -> [w300 _]
          tunnel: [w301 w307] -> w292
          frame No Error {
            n125 = Unbundle By Name(w303) -> ("Ls1Shutter"=w304:refnum<vi>, "Ls1 Status Ind"=w299:refnum<vi>)
            n126 = case shown="False" w300 {
              selector: w300 -> [w305 _]
              tunnel: w299 -> [w306 _]
              frame False {
                n127 = property class="Bool"(reference=w306, "Value"=w305) -> ()  [unwired: 1 in, 2 out]
              }
              frame True {
              }
            }
            n128 = property class="Bool (strict)"(reference=w304, error in=w302, "Value"=w300) -> (error out=w301:errorcluster)  [unwired: 1 out]
          }
          frame Error {
          }
        }
        n129 = Build Array(w292) -> (w293:errorcluster[])
      }
      frame "Update Laser Note" {
        n130 = Unbundle By Name(w314) -> ("Ls1 Note"=w313:refnum<vi>)
        n131 = Index Array(array=w312) -> (element=w311:string)  [unwired: 1 in]
        n132 = property class="Str"(reference=w313, "Value"=w311) -> ()  [unwired: 1 in, 2 out]
        n133 = Build Array(w309) -> (w308:errorcluster[])
      }
      frame "Close" {
        w317 = T5."Enabled" ("Disabled")
        w341 = FALSE ("Value")
        # "#NOTE\ncheck where the wavelength value is being read \nfor display and calculations"
        # "#DISABLED"
        n134 = case shown="True" w315 {
          tunnel: ["Not available" ("Value") "Closing" ("Value")] -> w323
          frame False {
          }
          frame True {
          }
        }
        n135 = Unbundle By Name(w338) -> ("Ls1 wav top Ind"=w348:refnum<vi>, "Ls1 power top Ind"=w347:refnum<vi>, "Ls1 Mode"=w346:refnum<vi>, "Ls1Tuning Status"=w345:refnum<vi>, "Ls1 Faults"=w344:refnum<vi>, "Ls1 Conn. Status"=w324:refnum<vi>, "Ls1 Note"=w322:refnum<vi>)
        n136 = Unbundle By Name(w338) -> ("Ls1Shutter"=w320:refnum<vi>, "Confirm Wav"=w352:refnum<vi>, "Ls1 Wavelength"=w353:refnum<vi>, "Live Imaging"=w351:refnum<vi>, "AOL Z Stack"=w350:refnum<vi>, "Motor Z Stack"=w349:refnum<vi>)
        n137 = Unbundle By Name(w338) -> ("Ls1 Connection"=w343:refnum<vi>, "Ls1 Status Ind"=w342:refnum<vi>)
        n138 = property class="Bool (strict)"(reference=w320, "DisabledEnum"=T5."Disabled and Grayed Out" ("Disabled")) -> (error out=w318:errorcluster)  [unwired: 1 in, 1 out]
        n139 = property class="DigNum (strict)"(reference=w353, "DisabledEnum"=w317) -> (error out=w335:errorcluster)  [unwired: 1 in, 1 out]
        n140 = property class="Bool (strict)"(reference=w351, "DisabledEnum"=w317) -> (error out=w334:errorcluster)  [unwired: 1 in, 1 out]
        n141 = property class="Bool (strict)"(reference=w350, "DisabledEnum"=w317) -> (error out=w333:errorcluster)  [unwired: 1 in, 1 out]
        n142 = property class="Bool (strict)"(reference=w349, "DisabledEnum"=w317) -> (error out=w332:errorcluster)  [unwired: 1 in, 1 out]
        n143 = property class="Bool"(reference=w352, "DisabledEnum"=w317) -> (error out=w336:errorcluster)  [unwired: 1 in, 1 out]
        n144 = disable-structure shown="Enabled" {
          disable-tunnel: w348 -> [w356 _]
          frame Disabled {
            n145 = property class="Str" props=["Value"](reference=w356) -> ()  [unwired: 2 in, 2 out]
          }
          frame Enabled {
          }
        }
        n146 = property class="Str"(reference=w347, "Value"="") -> (error out=w331:errorcluster)  [unwired: 1 in, 1 out]
        n147 = property class="Str"(reference=w346, "Value"=w323) -> (error out=w330:errorcluster)  [unwired: 1 in, 1 out]
        n148 = property class="Str"(reference=w345, "Value"=w323) -> (error out=w329:errorcluster)  [unwired: 1 in, 1 out]
        n149 = property class="Str"(reference=w344, "Value"=w323) -> (error out=w328:errorcluster)  [unwired: 1 in, 1 out]
        n150 = property class="Str"(reference=w324, "Value"=w323) -> ()  [unwired: 1 in, 2 out]
        n151 = property class="Str"(reference=w322, "Value"="") -> ()  [unwired: 1 in, 2 out]
        n152 = property class="Bool (strict)"(reference=w343, "Value"=w341) -> (error out=w327:errorcluster)  [unwired: 1 in, 1 out]
        n153 = property class="Bool"(reference=w342, "Value"=w341) -> (reference out=w340:refnum<vi>)  [unwired: 1 in, 1 out]
        n154 = property class="Bool"(reference=w340, "DisabledEnum"=T5."Disabled and Grayed Out" ("Disabled")) -> (error out=w326:errorcluster)  [unwired: 1 in, 1 out]
        n155 = Build Array(w318, w336, w335, w334, w333, w332, w331, w330, w329, w328, w327, w326) -> (w325:errorcluster[])
      }
    }
  }
  "Read Wavelength" <- w3
  "Array" <- w1
  "Error out" <- "Error in"
